vi "Pre-Uninstall Custom Action.vi"() -> (0 "error out":errorcluster)   [LabVIEW 2021]
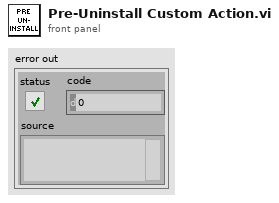
[diagram p1: front panel]
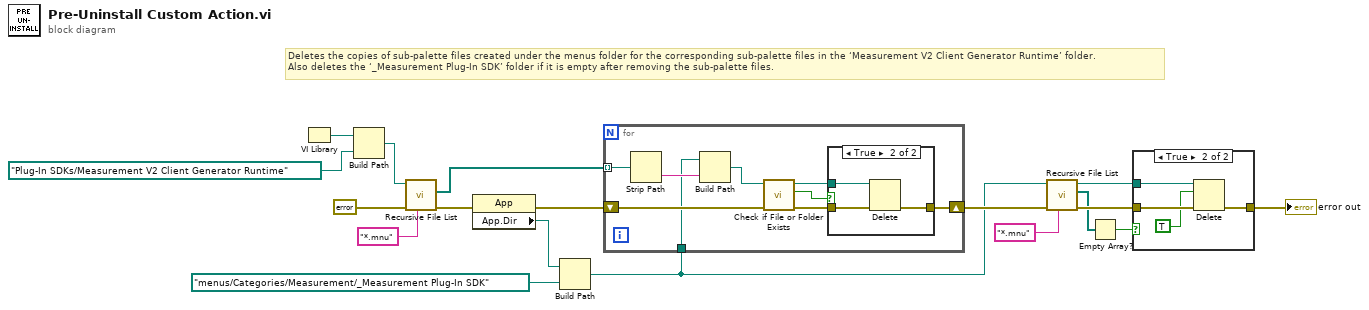
[diagram p0: block diagram]
diagram:
  # "Deletes the copies of sub-palette files created under the menus folder for the corresponding sub-palette files in the ‘Measurement V2 Client Generator Runtime’ folder.\nAlso deletes the ‘_Measurement Plug-In SDK’ folder if it is empty after removing the sub-palette files."
  n1 = VI Library() -> (path=w12:path)
  n2 = Build Path(base path=w12, name or relative path=path "Plug-In SDKs/Measurement V2 Client Generator Runtime") -> (appended path=w4:path)
  n3 = call <vilib>:"Recursive File List.vi"("pattern"="*.mnu", "error in (no error)"=errorcluster {"status"=FALSE, "code"=0, "source"=""}, "Folder Path"=w4) -> ("error out"=w14:errorcluster, "All Files in Dir"=w2:path[])  [unwired: 4 in, 3 out]
  n4 = property class="App"(error in=w14) -> (error out=w17:errorcluster, "App.Dir"=w16:path)  [unwired: 1 in, 1 out]
  n5 = Build Path(base path=w16, name or relative path=path "menus/Categories/Measurement/_Measurement Plug-In SDK") -> (appended path=w10:path)
  n6 = for {
    tunnel: w10 -> [w20]
    shift-right: [w21] -> w13
    shift-left: w17 -> [w27]
    tunnel: w2 -> [w19] mode=indexing
    n7 = Strip Path(path=w19) -> (name=w26:string)  [unwired: 1 out]
    n8 = Build Path(base path=w20, name or relative path=w26) -> (appended path=w25:path)
    n9 = call <vilib>:"Check if File or Folder Exists.vi"("error in (no error)"=w27, "path"=w25) -> ("error out"=w24:errorcluster, "file or folder exists?"=w23:bool, "dup path"=w22:path)  [unwired: 7 in]
    n10 = case shown="True" w23 {
      tunnel: [w28 w31] -> w21
      tunnel: w24 -> [w28 w30]
      tunnel: w22 -> [_ w29]
      frame False {
      }
      frame True {
        n11 = Delete(path (use dialog)=w29, error in=w30) -> (error out=w31:errorcluster)  [unwired: 3 in, 2 out]
      }
    }
  }
  n12 = call <vilib>:"Recursive File List.vi"("pattern"="*.mnu", "error in (no error)"=w13, "Folder Path"=w10) -> ("error out"=w11:errorcluster, "All Files in Dir"=w8:path[], "dup Folder Path"=w6:path)  [unwired: 4 in, 2 out]
  n13 = Empty Array?(array=w8) -> (empty?=w5:bool)
  n14 = case shown="True" w5 {
    tunnel: w11 -> [w32 w36]
    tunnel: [w32 w35] -> w7
    tunnel: w6 -> [_ w34]
    frame False {
    }
    frame True {
      n15 = Delete(path (use dialog)=w34, entire hierarchy (F)=TRUE, error in=w36) -> (error out=w35:errorcluster)  [unwired: 2 in, 2 out]
    }
  }
  "error out" <- w7
